vi "UKSupportMouseClickversion82[v2].vi"() -> (0 "Last Mouse Position:All Elements":cluster{"X":i32, "Y":i32}, 1 "Coords":T1)   [LabVIEW 2015]
uses:
  <vilib>/Utility/miscctls.llb/LVPoint32TypeDef.ctl
panel:
  in  "stop":bool
  out "Snap - Right":T2(plugin-control)
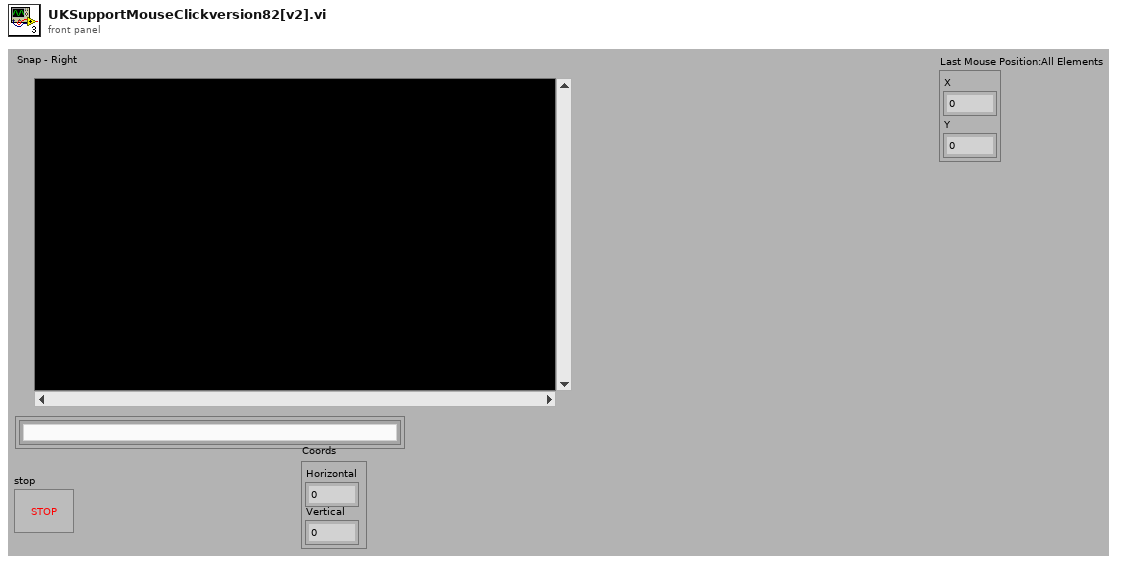
[diagram p1: front panel]
types:
  T1 = typedef "LVPoint32TypeDef.ctl" = cluster{"Horizontal":i32, "Vertical":i32}
  T2 = typedef "IMAQ Image.ctl" = refnum<image>
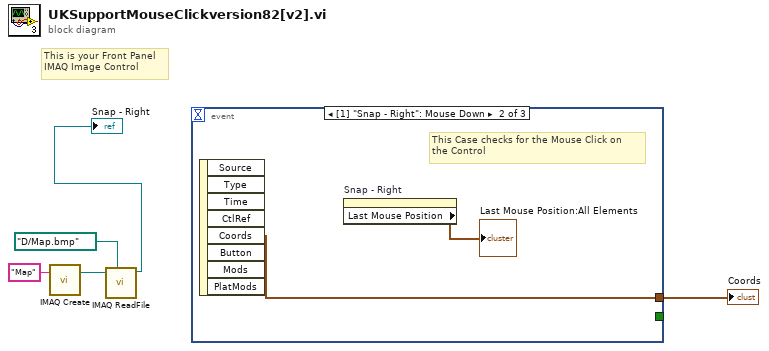
[diagram p0: block diagram]
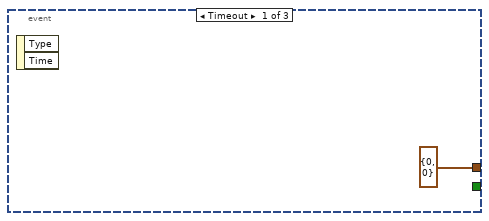
[diagram p2: hidden frame]
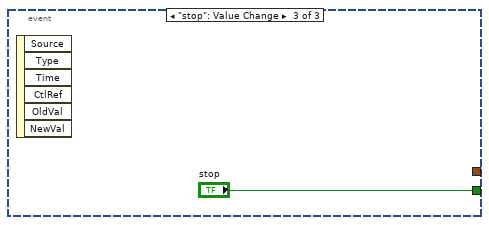
[diagram p3: hidden frame]
diagram:
  # "This is your Front Panel\nIMAQ Image Control"
  n1 = call "IMAQ Create"("Image Name"="Map") -> ("New Image"=w3:T2)  [unwired: 4 in, 1 out]
  n2 = call "IMAQ ReadFile"("File Path"=path "D:/Map.bmp", "Image"=w3) -> ("Image Out"=→"Snap - Right":T2)  [unwired: 5 in, 4 out]
  n3 = event shown="[1] \"Snap - Right\": Mouse Down" {
    selector: _ -> [_ _ _]
    dyn-events: _ -> [_ _ _]
    timeout: _ -> [_ _ _]
    tunnel: [T1 {"Horizontal"=0, "Vertical"=0} ("Coords") w8 _] -> w5
    tunnel: [_ _ "stop"] -> _
    event Timeout {
      n4 = event-data() -> ()  [unwired: 3 out]
    }
    event "Snap - Right": Mouse Down {
      # "This Case checks for the Mouse Click on\nthe Control"
      n5 = event-data() -> ("Coords"=w8:T1)  [unwired: 8 out]
      n6 = property on="Snap - Right" class="ImageControl"() -> ("Last Mouse Position"=→"Last Mouse Position:All Elements":cluster{"X":i32, "Y":i32})  [unwired: 2 in, 2 out]
    }
    event "stop": Value Change {
      n7 = event-data() -> ()  [unwired: 7 out]
    }
  }
  "Coords" <- w5
